vi "Write T start_stop.vi"(9 "T_heat_stop":u32=300, 10 "T_heat_start":u32=300, 11 "HE_ZM_state in":refnum<class "HE_ZM_state.lvclass">) -> (3 "HE_ZM_state out":refnum<class "HE_ZM_state.lvclass">)   [LabVIEW 2019, in "Heating.lvlib" / "HE_ZM_state.lvclass"]
uses:
  HE_ZM_state.lvclass
  HE_ZM_state.lvclass/HE_ZM_state.ctl
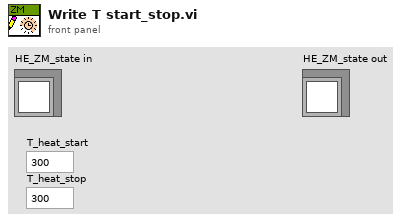
[diagram p1: front panel]
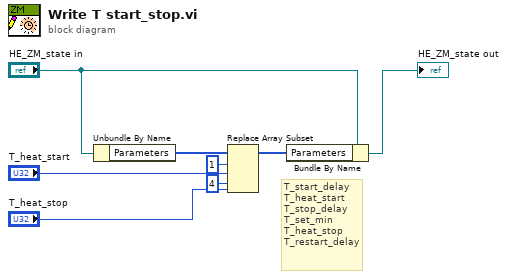
[diagram p0: block diagram]
diagram:
  # "T_start_delay\nT_heat_start\nT_stop_delay\nT_set_min\nT_heat_stop\nT_restart_delay"
  n1 = Unbundle By Name("HE_ZM_state in") -> ("Parameters"=w6:u32[])
  n2 = Replace Array Subset(array=w6, new element #1="T_heat_start", index #1=1 ("index"), new element #2="T_heat_stop", index #2=4 ("index")) -> (w5:u32[])
  n3 = Bundle By Name(cluster="HE_ZM_state in", "Parameters"=w5) -> (→"HE_ZM_state out":refnum<class "HE_ZM_state.lvclass">)
